vi "ITX Folder to PG.vi"(8 "error in (no error)":errorcluster, 11 "Folder Path":path) -> (0 "error out":errorcluster)   [LabVIEW 2016]
uses:
  Data/Data.lvclass
panel:
  in  "stop":bool
  in  "Additional Notes?":string
  out "Elapsed Time (s)":dbl
  out "Numeric":i32
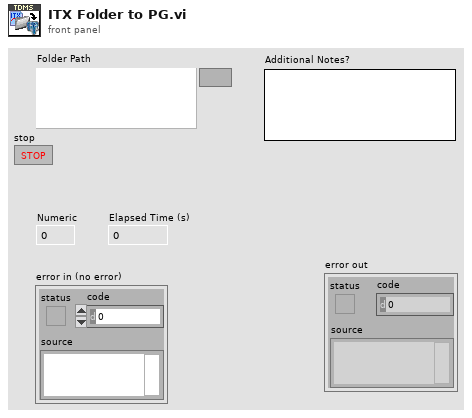
[diagram p1: front panel]
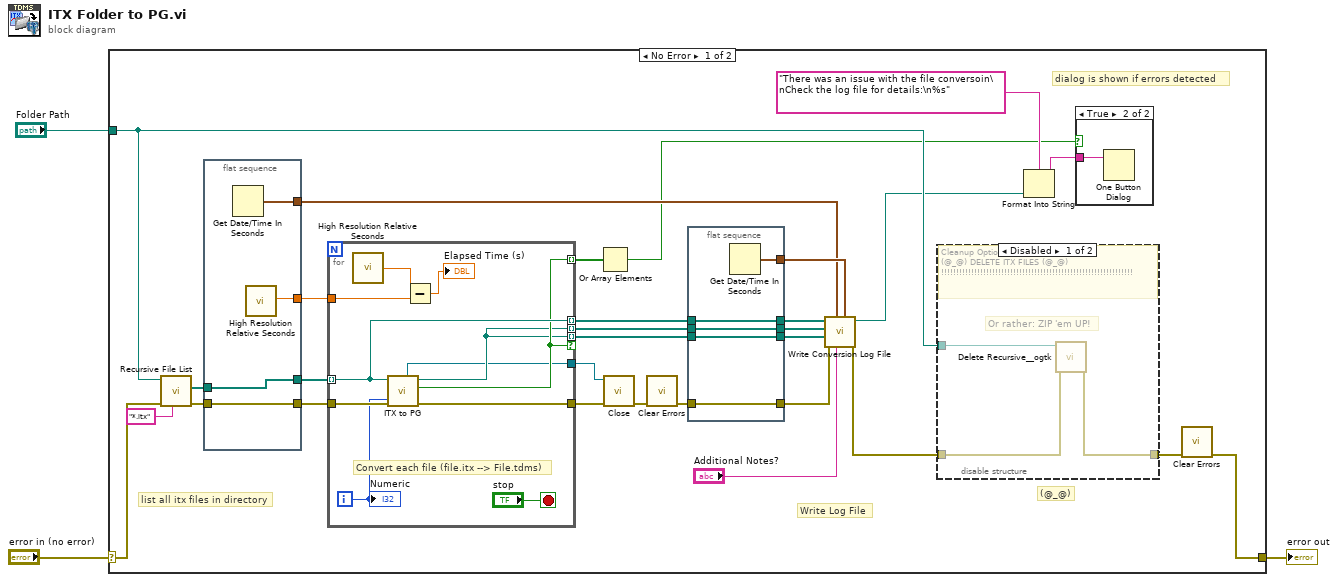
[diagram p0: block diagram]
diagram:
  n1 = case shown="No Error" "error in (no error)" {
    selector: "error in (no error)" -> [w32 w59]
    tunnel: [w9 w59] -> w2
    tunnel: "Folder Path" -> [w12 _]
    frame No Error {
      # "(@_@)"
      # "dialog is shown if errors detected"
      # "list all itx files in directory"
      # "Write Log File"
      n2 = call <vilib>:"Recursive File List.vi"("pattern"="*.itx", "error in (no error)"=w32, "Folder Path"=w12) -> ("error out"=w28:errorcluster, "All Files in Dir"=w27:path[])  [unwired: 4 in, 3 out]
      n3 = flat-sequence {
        tunnel: [w42] -> w31
        tunnel: [w41] -> w29
        tunnel: w28 -> [w41]
        tunnel: w27 -> [w40]
        tunnel: [w40] -> w26
        tunnel: [w39] -> w15
        frame #0 {
          n4 = Get Date/Time In Seconds() -> (seconds since 1Jan1904=w39:timestamp)
          n5 = call <vilib>:"High Resolution Relative Seconds.vi"() -> ("relative seconds"=w42:dbl)
        }
      }
      n6 = for {
        tunnel: w26 -> [w53] mode=indexing
        tunnel: w29 -> [w57]
        tunnel: [w56] -> w6
        tunnel: w31 -> [w54]
        tunnel: [w50] -> w22 mode=indexing if=w52
        tunnel: [w50] -> w24 mode=indexing
        tunnel: [w53] -> w25 mode=indexing
        tunnel: [w52] -> w30 mode=indexing
        tunnel: [w49] -> w7
        i -> [w48]
        stop <- "stop" stop-if-true
        # "Convert each file (file.itx --> File.tdms)"
        n7 = call <vilib>:"High Resolution Relative Seconds.vi"() -> ("relative seconds"=w55:dbl)
        n8 = call "ITX to PG.vi"("Numeric"=w48, "error in (no error)"=w57, "Path"=w53) -> ("error out"=w56:errorcluster, "Not Equal?"=w52:bool, "Path out"=w50:path, "Data out"=w49:refnum<class "Data.lvclass">)  [unwired: 5 in]
        n9 = Subtract(x=w55, y=w54) -> (x-y=→"Elapsed Time (s)":dbl)
        "Numeric" <- w48
      }
      n10 = Or Array Elements(Boolean array=w30) -> (logical OR=w4:bool)
      n11 = call-dynamic "Close.vi"("error in (no error)"=w6, "Data in"=w7) -> ("error out"=w5:errorcluster)  [unwired: 8 in, 1 out]
      n12 = call <vilib>:"Clear Errors.vi"("error in (no error)"=w5) -> ("error out"=w10:errorcluster)  [unwired: 5 in, 1 out]
      n13 = flat-sequence {
        tunnel: w25 -> [w37]
        tunnel: [w38] -> w17
        tunnel: w24 -> [w38]
        tunnel: [w37] -> w18
        tunnel: [w36] -> w23
        tunnel: w22 -> [w36]
        tunnel: w10 -> [w35]
        tunnel: [w35] -> w13
        tunnel: [w34] -> w21
        frame #0 {
          n14 = Get Date/Time In Seconds() -> (seconds since 1Jan1904=w34:timestamp)
        }
      }
      n15 = call "Write Conversion Log File.vi"("End time"=w21, "Additional Notes?"="Additional Notes?", "Start time"=w15, "error in (no error)"=w13, "Failed Converted Files"=w23, "Converted Files"=w17, "Original Files"=w18) -> ("error out"=w14:errorcluster, "Log File Path"=w11:path)  [unwired: 3 in]
      n16 = disable-structure shown="Disabled" {
        disable-tunnel: w14 -> [w45 w46]
        disable-tunnel: [w44 w46] -> w16
        disable-tunnel: w12 -> [w43 _]
        frame Disabled {
          # "Or rather: ZIP 'em UP!"
          # "Cleanup Option:\n(@_@) DELETE ITX FILES (@_@)\n!!!!!!!!!!!!!!!!!!!!!!!!!!!!!!!!!!!!!!!!!!!!!!!!!!!!!!!!!!!!!!!!"
          n17 = call <userlib>:"Delete Recursive__ogtk.vi"("error in (no error)"=w45, "Path"=w43) -> ("error out"=w44:errorcluster)  [unwired: 8 in, 1 out]
        }
        frame Enabled {
        }
      }
      n18 = Format Into String(format string="There was an issue with the file conversoin\nCheck the log file for details:\n%s", w11) -> (resulting string=w20:string)  [unwired: 2 in, 1 out]
      n19 = case shown="True" w4 {
        tunnel: w20 -> [_ w58]
        frame False {
        }
        frame True {
          n20 = One Button Dialog(message=w58) -> ()  [unwired: 1 in, 1 out]
        }
      }
      n21 = call <vilib>:"Clear Errors.vi"("error in (no error)"=w16) -> ("error out"=w9:errorcluster)  [unwired: 5 in, 1 out]
    }
    frame Error {
    }
  }
  "error out" <- w2
